vi "Configure TV Trigger Source [TV] Core.vi"(0 "IVI_Scope in":refnum<class "IVI_Scope.lvclass">, 1 "trigger source (\"CHANNEL1\")":string(combo)="CHANNEL1", 2 "tv event (Field 1)":i32(ring)=1 items=["Field 1"=1, "Field 2"=2, "Any Field"=3, "Any Line"=4, "Line Number"=5], 3 "tv trigger polarity (Positive)":i32(ring)=1 items=["Positive"=1, "Negative"=2], 4 "tv signal format (NTSC)":i32(ring)=1 items=["NTSC"=1, "PAL"=2, "SECAM"=3], 5 "error in (no error)":errorcluster) -> (14 "IVI_Scope out":refnum<class "IVI_Scope.lvclass">, 19 "error out":errorcluster)   [LabVIEW 2013, in "IVI_Scope.lvlib" / "IVI_Scope.lvclass"]
doc: "This VI configures the oscilloscope for TV triggering. It configures the TV signal format, the event and the signal polarity."
uses:
  IVI_Scope.lvclass
  IVI_Scope.lvclass/IVI_Scope.ctl
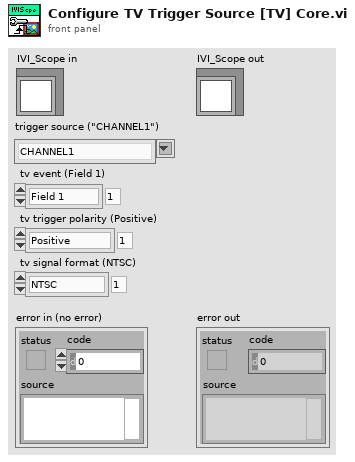
[diagram p1: front panel]
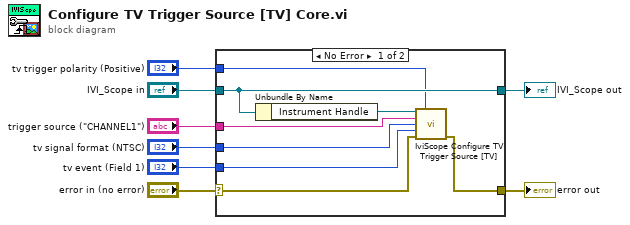
[diagram p0: block diagram]
diagram:
  n1 = case shown="No Error" "error in (no error)" {
    selector: "error in (no error)" -> [w16 w18]
    tunnel: [w15 w18] -> w7
    tunnel: [w14 w17] -> w5
    tunnel: "IVI_Scope in" -> [w14 w17]
    tunnel: "trigger source (\"CHANNEL1\")" -> [w12 _]
    tunnel: "tv signal format (NTSC)" -> [w11 _]
    tunnel: "tv event (Field 1)" -> [w10 _]
    tunnel: "tv trigger polarity (Positive)" -> [w9 _]
    frame No Error {
      n2 = Unbundle By Name(w14) -> ("Instrument Handle"=w13:refnum<k15>)
      n3 = call <vilib>:"IviScope Configure TV Trigger Source [TV].vi"("instrument handle"=w13, "tv trigger polarity (Positive)"=w9, "trigger source (\"CHANNEL1\")"=w12, "tv signal format (NTSC)"=w11, "tv event (Field 1)"=w10, "error in (no error)"=w16) -> ("error out"=w15:errorcluster)  [unwired: 8 in, 1 out]
    }
    frame Error {
    }
  }
  "error out" <- w7
  "IVI_Scope out" <- w5
